vi "AndorPhysikInstrumenteInitialisiation.vi"(7 "reference":refnum<vi>, 8 "error in (no error)":errorcluster, 9 "reference 3":refnum<vi>, 10 "reference 2":refnum<vi>, 11 "Pi":i32) -> (0 "error out":errorcluster, 3 "Device List":T1(array[cluster]))   [LabVIEW 2013]
uses:
  Variables/GlobalConAxisPI.vi
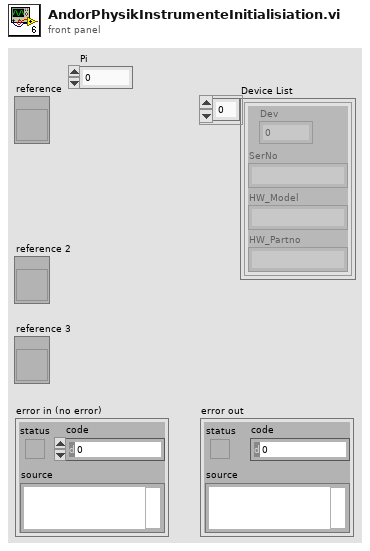
[diagram p1: front panel]
types:
  T1 = cluster{"Dev":i32, "SerNo":string, "HW_Model":string, "HW_Partno":string}[]
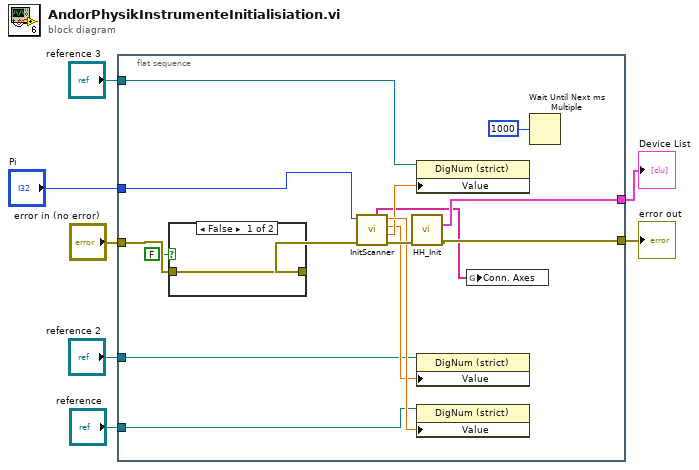
[diagram p0: block diagram]
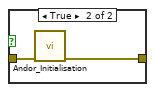
[diagram p2: hidden frame]
diagram:
  n1 = flat-sequence {
    tunnel: [w22] -> w5
    tunnel: "error in (no error)" -> [w17]
    tunnel: [w11] -> w7
    tunnel: "reference" -> [w14]
    tunnel: "reference 2" -> [w13]
    tunnel: "reference 3" -> [w12]
    tunnel: "Pi" -> [w10]
    frame #0 {
      n2 = case shown="False" FALSE {
        tunnel: w17 -> [w23 w25]
        tunnel: [w23 w24] -> w16
        frame False {
        }
        frame True {
          n3 = call "Andor_Initialisation.vi"("error in (no error)"=w25) -> ("error out"=w24:errorcluster)  [unwired: 10 in]
        }
      }
      n4 = call "InitScanner.vi"("error in (no error)"=w16, "PI SystemNumber"=w10) -> ("error out"=w21:errorcluster, "z-position"=w19:dbl, "y-position"=w18:dbl, "x-position"=w20:dbl, "Conn. Axes"=w9:string[])  [unwired: 5 in]
      n5 = call "HH_Init.vi"("error in (no error)"=w21) -> ("Device List"=w22:T1, "error out"=w11:errorcluster)  [unwired: 12 in, 1 out]
      n6 = property class="DigNum (strict)"(reference=w12, "Value"=w19) -> ()  [unwired: 1 in, 2 out]
      n7 = property class="DigNum (strict)"(reference=w13, "Value"=w18) -> ()  [unwired: 1 in, 2 out]
      n8 = property class="DigNum (strict)"(reference=w14, "Value"=w20) -> ()  [unwired: 1 in, 2 out]
      n9 = global write "GlobalConAxisPI.vi" "Conn. Axes"(w9) -> ()
      n10 = Wait Until Next ms Multiple(millisecond multiple=u32 1000) -> ()  [unwired: 1 out]
    }
  }
  "error out" <- w7
  "Device List" <- w5
